vi "AFT Linear Prediction (Array).vi"(6 "step size":dbl=-1.0, 7 "reset? (F)":bool, 8 "error in (no error)":errorcluster, 10 "signal":dbl[](array[numeric]), 11 "adaptive filter in":refnum<k20>) -> (0 "error out":errorcluster, 1 "prediction error":dbl[](array[numeric]), 3 "adaptive filter out":refnum<k20>, 4 "AR coefficients":dbl[](array[numeric]))   [LabVIEW 2017, in "NI_AdaptiveFilter.lvlib"]
doc: "Performs adaptive linear prediction by estimating the autoregressive (AR) model of an input signal. Wire data to the <B>signal</B> input to determine the polymorphic instance to use or manually select the instance."
uses:
  <vilib>/addons/Adaptive Filters/NI_AdaptiveFilter.lvlib
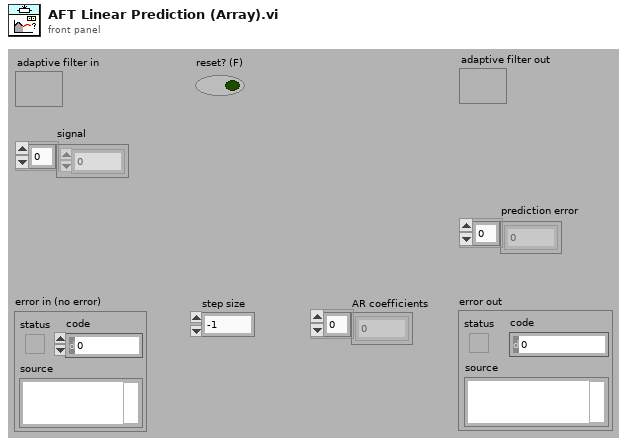
[diagram p1: front panel]
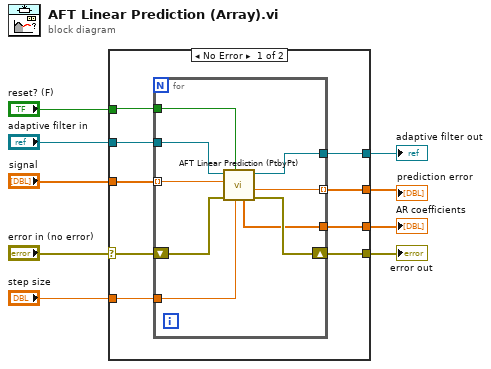
[diagram p0: block diagram]
diagram:
  n1 = case shown="No Error" "error in (no error)" {
    selector: "error in (no error)" -> [w15 w29]
    tunnel: "adaptive filter in" -> [w17 w28]
    tunnel: [w12 w28] -> w8
    tunnel: "signal" -> [w18 _]
    tunnel: [w11 w29] -> w6
    tunnel: "reset? (F)" -> [w16 _]
    tunnel: "step size" -> [w14 _]
    tunnel: [w13 _] -> w3
    tunnel: [w10 _] -> w1
    frame No Error {
      n2 = for {
        tunnel: w18 -> [w27] mode=indexing
        tunnel: w17 -> [w26]
        tunnel: w16 -> [w25]
        shift-right: [w23] -> w11
        shift-left: w15 -> [w24]
        tunnel: w14 -> [w22]
        tunnel: [w21] -> w13
        tunnel: [w20] -> w12
        tunnel: [w19] -> w10 mode=indexing
        n3 = call <vilib>:"AFT Linear Prediction (PtbyPt).vi"("step size"=w22, "reset? (F)"=w25, "error in (no error)"=w24, "signal"=w27, "adaptive filter in"=w26) -> ("error out"=w23:errorcluster, "prediction error"=w19:dbl, "adaptive filter out"=w20:refnum<k20>, "AR coefficients"=w21:dbl[])  [unwired: 3 out]
      }
    }
    frame Error {
    }
  }
  "adaptive filter out" <- w8
  "error out" <- w6
  "AR coefficients" <- w3
  "prediction error" <- w1
